vi "Stop.vi"(8 "error in (no error)":errorcluster, 10 "Message in":refnum<class "StopMessage.lvclass">, 11 "Galvo in":refnum<class "InVivo_ImagingModeSPIM.lvclass">) -> (0 "error out":errorcluster, 3 "Galvo out":refnum<class "InVivo_ImagingModeSPIM.lvclass">)   [LabVIEW 2012, in "InVivo_ImagingModeSPIM.lvclass"]
doc: "This member function is called when the statemachine in the run.vi receives an 'stop' command. It relays the message to all observers of the component.\n\nOverride this member function in your derived class if you need additional stop functionality (but don't forget to call the parent method)."
uses:
  InVivo_ImagingModeSPIM.lvclass
  <vilib>/Distrio/Murmex/StopMessage/StopMessage.lvclass
  <vilib>/Distrio/Murmex/Murmex/Murmex.lvclass
  InVivo_ImagingModeSPIM.lvclass/InVivo_ImagingModeSPIM.ctl
panel:
  # "This method is called when the STOP\ntrigger is sent. \n\nOverride this method when your component needs to\nrespond to this trigger. \n\nCall parent for proper implementation"
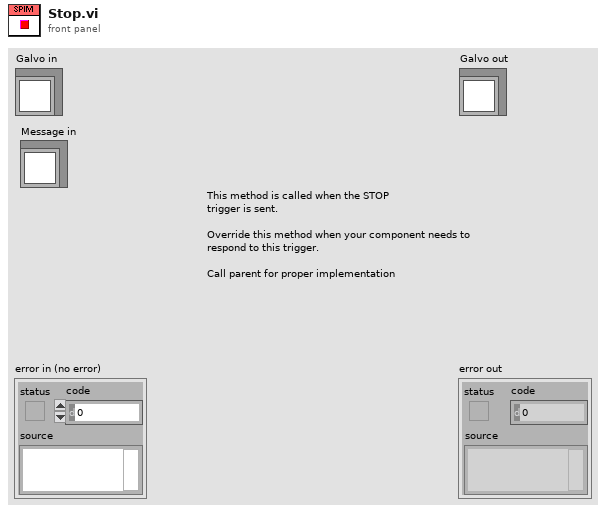
[diagram p1: front panel]
types:
  T1 = enum8{"Enabled", "Disabled", "Disabled and Grayed Out"}
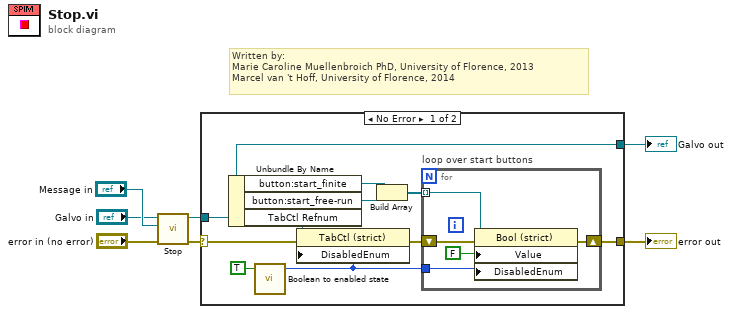
[diagram p0: block diagram]
diagram:
  # "Written by:\nMarie Caroline Muellenbroich PhD, University of Florence, 2013 \nMarcel van 't Hoff, University of Florence, 2014"
  n1 = call-parent "Stop.vi"("error in (no error)"="error in (no error)", "Message in"="Message in", "Murmex in"="Galvo in") -> ("error out"=w4:errorcluster, "Murmex out"=w3:refnum<class "InVivo_ImagingModeSPIM.lvclass">)  [unwired: 7 in]
  n2 = case shown="No Error" w4 {
    selector: w4 -> [w10 w23]
    tunnel: w3 -> [w17 w24]
    tunnel: [w17 w24] -> w2
    tunnel: [w13 w23] -> w1
    frame No Error {
      n3 = Unbundle By Name(w17) -> ("button:start_finite"=w16:refnum<vi>, "button:start_free-run"=w15:refnum<vi>, "TabCtl Refnum"=w11:refnum<vi>)
      n4 = call <vilib>:"Boolean to enabled state.vi"("boolean in"=TRUE) -> ("enabled status out"=w8:T1)  [unwired: 4 in]
      n5 = property class="TabCtl (strict)"(reference=w11, error in=w10, "DisabledEnum"=w8) -> (error out=w9:errorcluster)  [unwired: 1 out]
      n6 = Build Array(w16, w15) -> (w14:refnum<vi>[])
      n7 = for "loop over start buttons" {
        tunnel: w14 -> [w22] mode=indexing
        shift-right: [w20] -> w13
        shift-left: w9 -> [w21]
        tunnel: w8 -> [w18]
        n8 = property class="Bool (strict)"(reference=w22, error in=w21, "Value"=FALSE, "DisabledEnum"=w18) -> (error out=w20:errorcluster)  [unwired: 1 out]
      }
    }
    frame Error {
    }
  }
  "error out" <- w1
  "Galvo out" <- w2
